vi "DCC_get_gain_HV_limit.vi"(7 "Limit ID":i16, 8 "Error In":errorcluster, 9 "Gain":i16 min=0 max=100, 10 "Module No":i16, 11 "DLL Path":path) -> (0 "Error Out":errorcluster, 1 "Gain":i16 min=0 max=100, 2 "Module No":i16, 3 "DLL Path":path, 5 "Limit ID":i16)   [LabVIEW 2019]
doc: "The \"DCC_get_gain_HV_limit\" function reads the current value from the EEPROM of the DCC module specified by \"Module No\".\nDepending on the \"Lim ID\" the connector 1 or connector 3 gain HV will be read\nConnector 1: Lim ID=0 ; Connector 3: Lim ID=1).\n\nOctober 2018\nFrank Quadt & Stefan Smietana\ninfo@becker-hickl.com"
panel:
  # "(c) 2021 Becker & Hickl GmbH\n     All Rights Reserved."
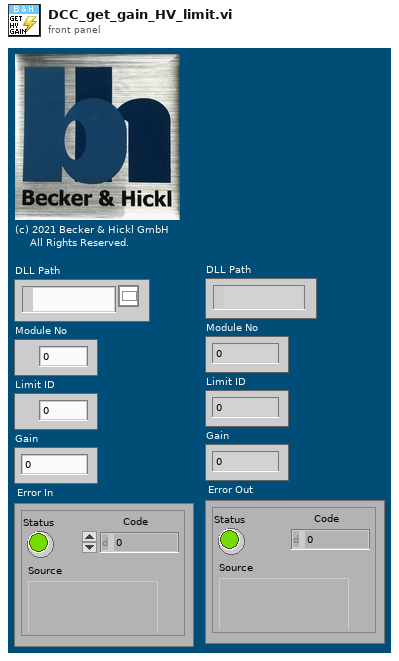
[diagram p1: front panel]
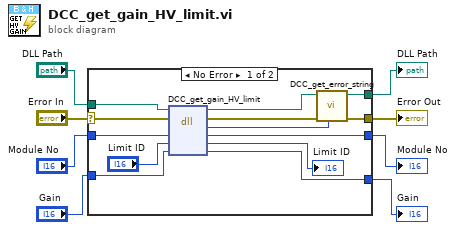
[diagram p0: block diagram]
diagram:
  n1 = case shown="No Error" "Error In" {
    selector: "Error In" -> [w21 w24]
    tunnel: [w16 w25] -> w7
    tunnel: "DLL Path" -> [w19 w25]
    tunnel: [w18 w23] -> w5
    tunnel: "Module No" -> [w17 w23]
    tunnel: [w13 w24] -> w3
    tunnel: "Gain" -> [w10 w22]
    tunnel: [w9 w22] -> w1
    frame No Error {
      n2 = dll-call lib="C:/Program Files/BH/DCC/DLL/dcc32.dll" fn="DCC_get_gain_HV_limit"(path in=w19, error in=w21, "ModuleNo"=w17, "LimitID"="Limit ID", "Gain"=w10) -> (path out=w20:path, error out=w14:errorcluster, "return type"=w15:i16, "ModuleNo"=w18:i16, "LimitID"=→"Limit ID":i16, "Gain"=w9:i16)  [unwired: 1 in]
      n3 = call "DCC_get_error_string.vi"("Error ID"=w15, "Error In"=w14, "DLL Path"=w20) -> ("Error Out"=w13:errorcluster, "DLL Path"=w16:path)  [unwired: 6 in, 1 out]
    }
    frame Error {
    }
  }
  "Error Out" <- w3
  "DLL Path" <- w7
  "Module No" <- w5
  "Gain" <- w1
